vi "Test Deserialize Clusters.vi"(8 "error in (no error)":errorcluster) -> (0 "error out":errorcluster)   [LabVIEW 2013]
uses:
  src/Serializer/JSON Serializer/JSON Serializer.lvclass
  src/Deserializer/JSON Deserializer/JSON Deserializer.lvclass
  <vilib>/addons/_JKI Toolkits/Caraya/classes/Test/Test.lvclass
  <vilib>/addons/_JKI Toolkits/Caraya/classes/Assert/Assert.lvclass
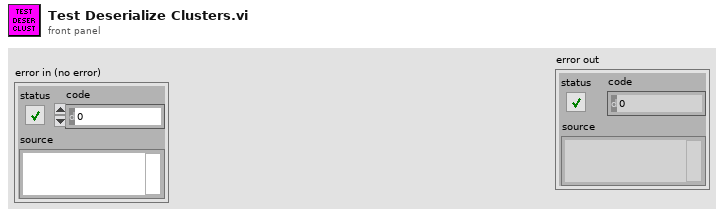
[diagram p1: front panel]
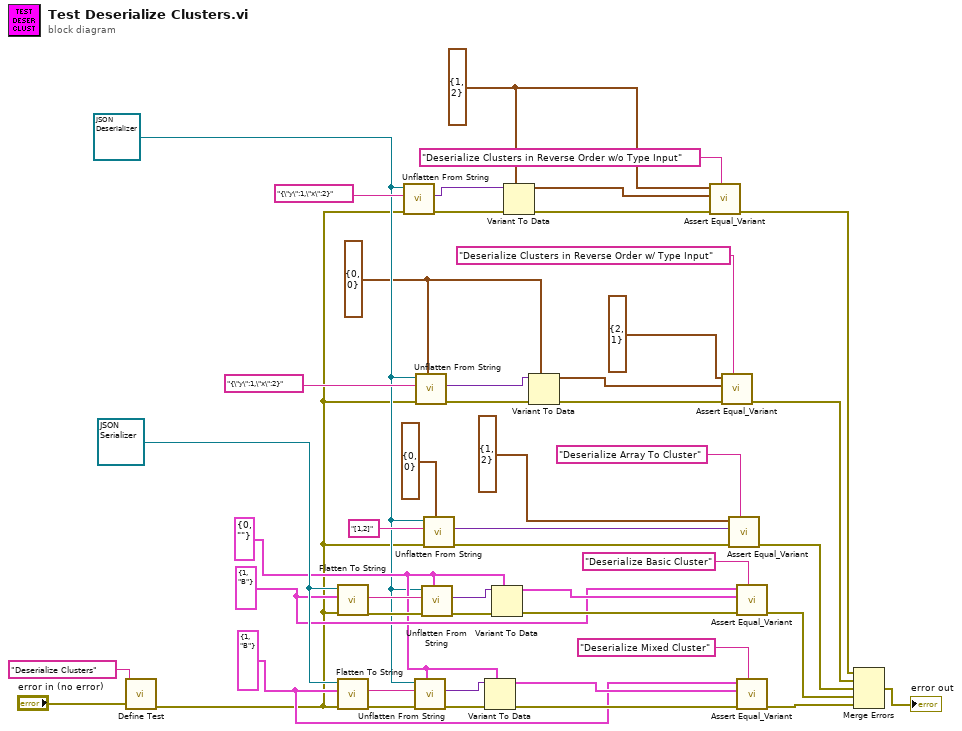
[diagram p0: block diagram]
diagram:
  w11 = cluster{"x":i32, "y":i32} {"x"=1, "y"=2}
  w4 = cluster{"x":i32, "y":i32} {"x"=0, "y"=0}
  w20 = cluster{"a":i32, "b":string} {"a"=0, "b"=""}
  w31 = cluster{"a":i32, string} {"a"=1, "B"}
  w22 = cluster{"a":i32, "b":string} {"a"=1, "b"="B"}
  w16 = refnum<class "JSON Deserializer.lvclass"> refnum ("Deserializer in")
  w30 = refnum<class "JSON Serializer.lvclass"> refnum ("JKI JSON Serialization.lvlib:JSON Serializer.lvclass")
  n1 = call <vilib>:"Define Test.vi"("error in (no error)"="error in (no error)", "Label (VI Title)"="Deserialize Clusters") -> ("error out"=w15:errorcluster)  [unwired: 9 in]
  n2 = call-dynamic "Flatten To String.vi"("error in (no error)"=w15, "Variant"=w22, "JSON Serializer in"=w30) -> ("error out"=w42:errorcluster, "String"=w41:string)  [unwired: 6 in, 1 out]
  n3 = call-dynamic "Flatten To String.vi"("error in (no error)"=w15, "Variant"=w31, "JSON Serializer in"=w30) -> ("error out"=w35:errorcluster, "String"=w34:string)  [unwired: 6 in, 1 out]
  n4 = call-dynamic "Unflatten From String.vi"("error in (no error)"=w15, "String"="{\"y\":1,\"x\":2}", "Deserializer in"=w16) -> ("error out"=w13:errorcluster, "Variant"=w12:variant)  [unwired: 6 in, 1 out]
  n5 = call-dynamic "Unflatten From String.vi"("Type and Defaults"=w20, "error in (no error)"=w35, "String"=w34, "Deserializer in"=w16) -> ("error out"=w37:errorcluster, "Variant"=w36:variant)  [unwired: 5 in, 1 out]
  n6 = call-dynamic "Unflatten From String.vi"("Type and Defaults"=w4, "error in (no error)"=w15, "String"="{\"y\":1,\"x\":2}", "Deserializer in"=w16) -> ("error out"=w2:errorcluster, "Variant"=w3:variant)  [unwired: 5 in, 1 out]
  n7 = call-dynamic "Unflatten From String.vi"("Type and Defaults"=w20, "error in (no error)"=w42, "String"=w41, "Deserializer in"=w16) -> ("error out"=w40:errorcluster, "Variant"=w21:variant)  [unwired: 5 in, 1 out]
  n8 = call-dynamic "Unflatten From String.vi"("Type and Defaults"=cluster{"x":i32, "y":i32} {"x"=0, "y"=0}, "error in (no error)"=w15, "String"="[1,2]", "Deserializer in"=w16) -> ("error out"=w25:errorcluster, "Variant"=w24:variant)  [unwired: 5 in, 1 out]
  n9 = Variant To Data(error in=w37, type=w20, Variant=w36) -> (data=w32:cluster{"a":i32, "b":string}, error out=w33:errorcluster)
  n10 = Variant To Data(error in=w40, type=w20, Variant=w21) -> (data=w39:cluster{"a":i32, "b":string}, error out=w38:errorcluster)
  n11 = Variant To Data(error in=w13, type=w11, Variant=w12) -> (data=w9:cluster{"x":i32, "y":i32}, error out=w10:errorcluster)
  n12 = Variant To Data(error in=w2, type=w4, Variant=w3) -> (data=w5:cluster{"x":i32, "y":i32}, error out=w1:errorcluster)
  n13 = call <vilib>:"Assert Equal_Variant.vi"("Label"="Deserialize Clusters in Reverse Order w/o Type Input", "error in (no error)"=w10, "Y"=w9, "X"=w11) -> ("error out"=w14:errorcluster)  [unwired: 7 in]
  n14 = call <vilib>:"Assert Equal_Variant.vi"("Label"="Deserialize Clusters in Reverse Order w/ Type Input", "error in (no error)"=w1, "Y"=w5, "X"=cluster{"x":i32, "y":i32} {"x"=2, "y"=1}) -> ("error out"=w18:errorcluster)  [unwired: 7 in]
  n15 = call <vilib>:"Assert Equal_Variant.vi"("Label"="Deserialize Array To Cluster", "error in (no error)"=w25, "Y"=w24, "X"=cluster{"x":i32, "y":i32} {"x"=1, "y"=2}) -> ("error out"=w26:errorcluster)  [unwired: 7 in]
  n16 = call <vilib>:"Assert Equal_Variant.vi"("Label"="Deserialize Basic Cluster", "error in (no error)"=w38, "Y"=w39, "X"=w22) -> ("error out"=w44:errorcluster)  [unwired: 7 in]
  n17 = call <vilib>:"Assert Equal_Variant.vi"("Label"="Deserialize Mixed Cluster", "error in (no error)"=w33, "Y"=w32, "X"=w31) -> ("error out"=w45:errorcluster)  [unwired: 7 in]
  n18 = Merge Errors(w14, w18, w26, w44, w45) -> (→"error out":errorcluster)
